vi "Pump 5 RT FIFO.vi"(0 "Data IN":u16[](array[numeric]), 1 "Mode":T1=enum."Delete", 7 "Buffer Size":i32=10, 9 "# of elements":i32=1, 11 "Error IN":errorcluster, 12 "Pause":bool) -> (4 "Data OUT":u16[][](array[numeric]), 15 "Error OUT":errorcluster)   [LabVIEW 2019]
uses:
  Real-Time/Controls/RT FIFO Mode.ctl
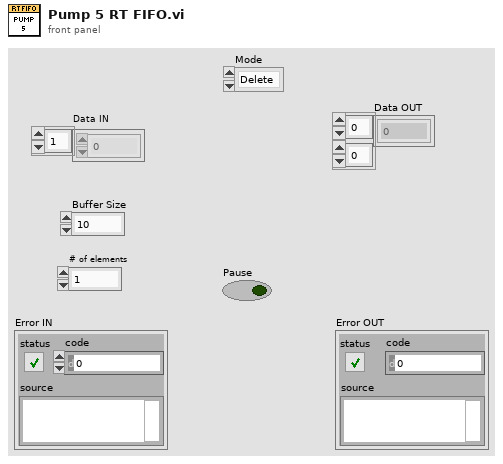
[diagram p1: front panel]
types:
  T1 = typedef "RT FIFO Mode.ctl" = enum16{"Create", "Write", "Read", "Delete"}
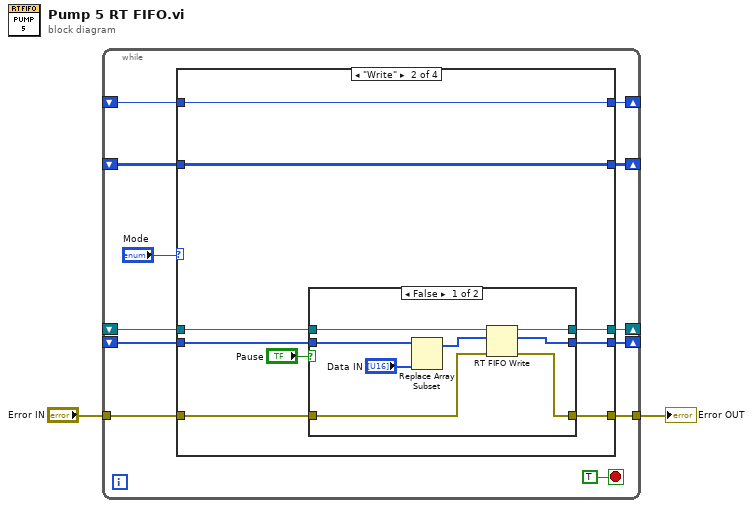
[diagram p0: block diagram]
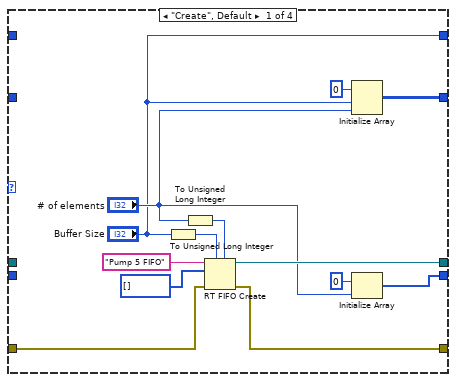
[diagram p2: hidden frame]
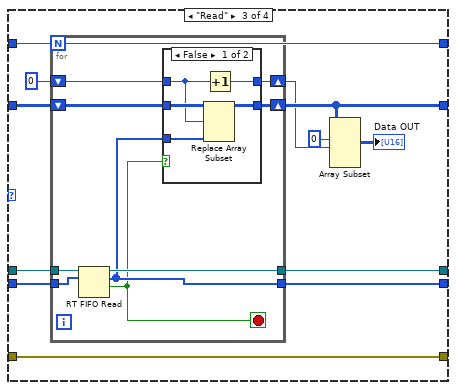
[diagram p4: hidden frame]
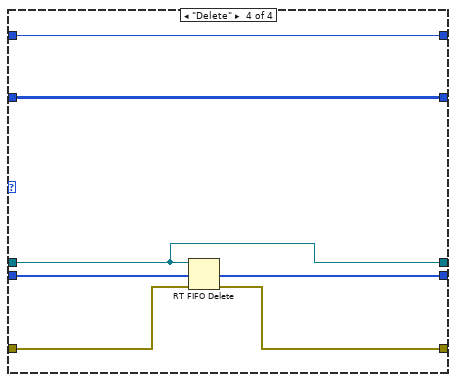
[diagram p6: hidden frame]
diagram:
  n1 = while {
    shift-right: [w12] -> _
    shift-left: _ -> [w11]
    tunnel: "Error IN" -> [w10]
    tunnel: [w9] -> w1
    shift-right: [w8] -> _
    shift-left: _ -> [w7]
    shift-right: [w6] -> _
    shift-left: _ -> [w5]
    shift-right: [w4] -> _
    shift-left: _ -> [w3]
    stop <- TRUE stop-if-true
    n2 = case shown="\"Write\"" "Mode" {
      tunnel: [w26 w35 w56 w80] -> w12
      tunnel: w11 -> [_ w36 w57 w80]
      tunnel: w10 -> [w22 w32 w58 w78]
      tunnel: [w21 w31 w58 w77] -> w9
      tunnel: [w23 w33 w54 w79] -> w8
      tunnel: w7 -> [_ w34 w55 w79]
      tunnel: [w16 w30 w51 w76] -> w6
      tunnel: w5 -> [_ w30 w52 w76]
      tunnel: ["Buffer Size" w29 w47 w75] -> w4
      tunnel: w3 -> [_ w29 w47 w75]
      frame "Create", Default {
        n3 = To Unsigned Long Integer(number="Buffer Size") -> (unsigned 32bit integer=w17:u32)
        n4 = To Unsigned Long Integer(number="# of elements") -> (unsigned 32bit integer=w20:u32)
        n5 = RT FIFO Create(0:"Pump 5 FIFO" ("name (unnamed)"), 1:u16[] [], 3:w22, 4:w17, 6:w20) -> (8:w26:refnum<k33>, 11:w21:errorcluster)  [unwired: 3 in, 1 out]
        n6 = Initialize Array(u16 0, "Buffer Size", "# of elements") -> (w16:u16[][])
        n7 = Initialize Array(u16 0, "# of elements") -> (w23:u16[])
      }
      frame "Write" {
        n8 = case shown="False" "Pause" {
          tunnel: w36 -> [w43 w46]
          tunnel: [w42 w46] -> w35
          tunnel: w34 -> [w41 w45]
          tunnel: [w39 w45] -> w33
          tunnel: w32 -> [w38 w44]
          tunnel: [w37 w44] -> w31
          frame False {
            n9 = Replace Array Subset(array=w41, new element="Data IN") -> (w39:u16[])  [unwired: 1 in]
            n10 = RT FIFO Write(0:w43, 1:w39, 3:w38) -> (8:w42:refnum<k33>, 11:w37:errorcluster)  [unwired: 2 in, 2 out]
          }
          frame True {
          }
        }
      }
      frame "Read" {
        n11 = for {
          N: w47 -> [_]
          tunnel: w57 -> [w67]
          tunnel: [w66] -> w56
          tunnel: w55 -> [w65]
          tunnel: [w60] -> w54
          shift-right: [w63] -> w49
          shift-left: 0 -> [w64]
          shift-right: [w61] -> w51
          shift-left: w52 -> [w62]
          stop <- w59 stop-if-true
          n12 = RT FIFO Read(0:w67, 1:w65) -> (8:w66:refnum<k33>, 9:w60:u16[], 10:w59:bool)  [unwired: 2 in, 2 out]
          n13 = case shown="False" w59 {
            tunnel: w64 -> [w69 w74]
            tunnel: [w72 w74] -> w63
            tunnel: w62 -> [w71 w73]
            tunnel: [w70 w73] -> w61
            tunnel: w60 -> [w68 _]
            frame False {
              n14 = Replace Array Subset(array=w71, new element=w68, index (row)=w69) -> (w70:u16[][])  [unwired: 1 in]
              n15 = Increment(x=w69) -> (x+1=w72:i32)
            }
            frame True {
            }
          }
        }
        n16 = Array Subset(array=w51, index (row)=0 ("index"), length (row)=w49) -> (→"Data OUT":u16[][])  [unwired: 2 in]
      }
      frame "Delete" {
        n17 = RT FIFO Delete(0:w80, 3:w78) -> (11:w77:errorcluster)  [unwired: 1 in]
      }
    }
  }
  "Error OUT" <- w1
